vi "Actualizacion Credito.vi"(8 "error in (no error)":errorcluster, 10 "Credito":dbl, 11 "Monedas in":refnum<class "Monedas.lvclass">) -> (0 "error out":errorcluster, 3 "Monedas out":refnum<class "Monedas.lvclass">)   [LabVIEW 2020, in "Monedas.lvlib" / "Monedas.lvclass"]
uses:
  Monedas.lvclass
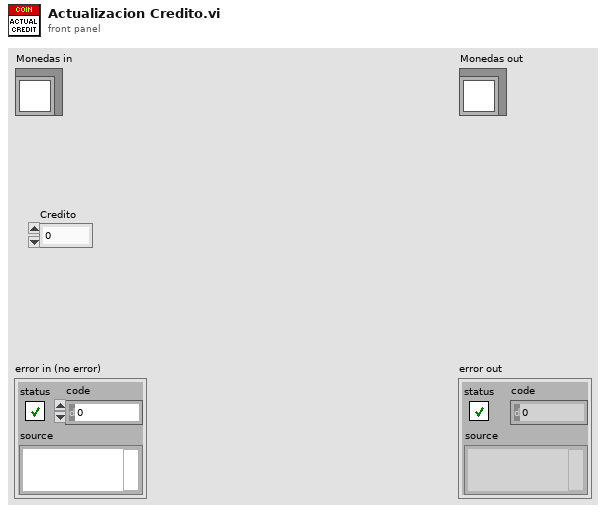
[diagram p1: front panel]
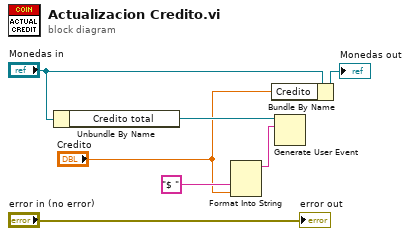
[diagram p0: block diagram]
diagram:
  n1 = Unbundle By Name("Monedas in") -> ("Credito total"=w4:refnum<user-event>)
  n2 = Format Into String("$ ", "Credito") -> (resulting string=w1:string)  [unwired: 3 in, 1 out]
  n3 = Bundle By Name(cluster="Monedas in", "Credito"="Credito") -> (→"Monedas out":refnum<class "Monedas.lvclass">)
  n4 = Generate User Event(user event=w4, event data cluster=w1) -> ()  [unwired: 2 in, 2 out]
  "error out" <- "error in (no error)"
